vi "PTSequencer.remove step.vi"(0 "i ref in":refnum<vi>, 2 "index":i32, 3 "ms timeout (10000)":i32=10000, 5 "error in (no error)":errorcluster) -> (14 "i ref out":refnum<vi>, 17 "timed out":bool, 19 "error out":errorcluster)   [LabVIEW 2014, in "PTSequencer.lvlib"]
uses:
  PTSequencer.lvlib
  _common/PTUtils/PTUtils.lvlib
  CSCore/CSSystem/CSSystemLib/CSSystemLib.lvlib
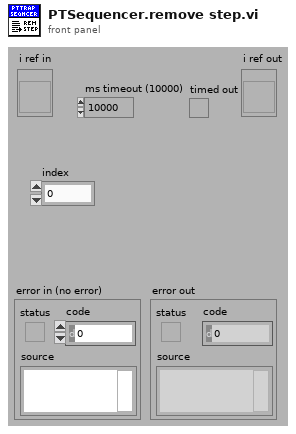
[diagram p1: front panel]
types:
  T1 = typedef "PTSequencer.lvlib/PTSequencer.i attribute.ctl" = cluster{"subsequence":bool, "mode":T2, "i step":i32, "nofLoops":i32, "i loop":i32, "Running":bool, "Paused":bool, "step done":bool, "loop done":bool, "seq done":bool, "DIM IDs":cluster{"step done":i32, "loop done":i32, "seq done":i32, "i step":i32, "i loop":i32}, "use stop conditions":bool, "stop conditions":T3[], "Step List":T5[], "DIM subsriptions":string[], "stop cond indexes":i32[], "step cond indexes":cluster{"step condition IDs":cluster{"step ID":i32, "condition ID":i32}[]}[], "Delay Start Time":timestamp, "status":string, "stopping":bool}
  T2 = typedef "PTSequencer.lvlib/PTSequencer.mode.ctl" = enum16{"single", "loop", "for loop"}
  T3 = typedef "PTSequencer.lvlib/PTSequencer.DIM service condition.ctl" = cluster{"DIM service":string, "descr":string, "nomValue":T4, "actValue":T4, "matched":bool, "DIM Status":cluster{"no link":bool, "quality":i32, "Time Stamp":timestamp}}
  T4 = typedef "CoreDefs.rawDataType.ctl" = i8[]
  T5 = typedef "PTSequencer.lvlib/PTSequencer.step.ctl" = cluster{"description":string, "object parameters":cluster{"object":string, "selector":string, "descriptor":string, "data":T4, "subsequence":bool, "call mode":enum16{"Simple DIM", "Synchronous"}, "data in":T4}, "result action":cluster{"check":bool, "passed":enum16{"Next", "Previous", "Repeat", "Jump"}, "failed":enum16{"Next", "Previous", "Repeat", "Jump"}, "jumpID_passed":i32, "jumpID_failed":i32}, "conditions":T3[], "fulfilled ":bool, "use delay":bool, "delay time (s)":dbl, "ID":i32}
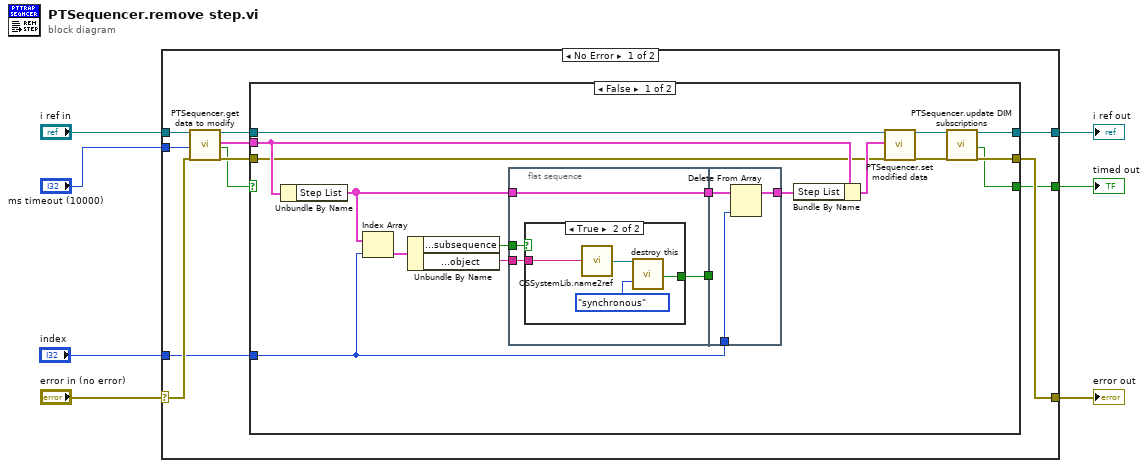
[diagram p0: block diagram]
diagram:
  n1 = case shown="No Error" "error in (no error)" {
    selector: "error in (no error)" -> [w15 w50]
    tunnel: "i ref in" -> [w18 w51]
    tunnel: [w9 w51] -> w6
    tunnel: "ms timeout (10000)" -> [w11 _]
    tunnel: [w8 _] -> w3
    tunnel: [w10 w50] -> w2
    tunnel: "index" -> [w12 _]
    frame No Error {
      n2 = call "PTSequencer.get data to modify.vi"("i ref in"=w18, "ms timeout (10000)"=w11, "error in (no error)"=w15) -> ("i ref out"=w17:refnum<vi>, "i attribute"=w16:T1, "timed out"=w13:bool, "error out"=w14:errorcluster)  [unwired: 13 in]
      n3 = case shown="False" w13 {
        selector: w13 -> [_ w47]
        tunnel: w17 -> [w35 w48]
        tunnel: [w23 w48] -> w9
        tunnel: w16 -> [w33 _]
        tunnel: w14 -> [w32 w49]
        tunnel: [w22 w49] -> w10
        tunnel: [w20 w47] -> w8
        tunnel: w12 -> [w25 _]
        frame False {
          n4 = Unbundle By Name(w33) -> ("Step List"=w28:T5[])
          n5 = Index Array(array=w28, index=w25) -> (element=w31:T5)
          n6 = Unbundle By Name(w31) -> ("object parameters.subsequence"=w30:bool, "object parameters.object"=w29:string)
          n7 = flat-sequence {
            tunnel: w30 -> [w39]
            tunnel: w29 -> [w38]
            tunnel: w28 -> [w37]
            tunnel: [w37] -> w27
            tunnel: [w36] -> w19
            tunnel: w27 -> [w46]
            tunnel: [w45] -> w26
            tunnel: w25 -> [w44]
            tunnel: w19 -> [_]
            frame #0 {
              n8 = case shown="True" w39 {
                tunnel: w38 -> [_ w43]
                tunnel: [_ w40] -> w36
                frame False {
                }
                frame True {
                  n9 = call "CSSystemLib.name2ref.vi"("name"=w43) -> ("obj refnum"=w42:refnum<vi>)
                  n10 = call "destroy this.vi"("i ref in"=w42, "CallType"=enum16{"simple", "synchronous", "asynchronous"}."synchronous") -> ("obj destroyed"=w40:bool)  [unwired: 17 in]
                }
              }
            }
            frame #1 {
              n11 = Delete From Array(array=w46, index=w44) -> (array with subset deleted=w45:T5[])  [unwired: 1 in, 1 out]
            }
          }
          n12 = Bundle By Name(cluster=w33, "Step List"=w26) -> (w34:T1)
          n13 = call "PTSequencer.set modified data.vi"("i ref in"=w35, "CLASS.i attribute"=w34, "error in (no error)"=w32) -> ("i ref out"=w24:refnum<vi>, "error out"=w21:errorcluster)  [unwired: 15 in]
          n14 = call "PTSequencer.update DIM subscriptions.vi"("i ref in"=w24, "error in"=w21) -> ("i ref out"=w23:refnum<vi>, "timed out"=w20:bool, "error out"=w22:errorcluster)  [unwired: 15 in]
        }
        frame True {
        }
      }
    }
    frame Error {
    }
  }
  "error out" <- w2
  "i ref out" <- w6
  "timed out" <- w3
